vi "Change Baud or Unit ID.vi"(7 "Unit ID (A)":string="A", 8 "error in":errorcluster, 9 "Change Unit Baud Rate":enum8{"2400", "9600", "19200", "38400"}(ring)=enum."19200", 10 "Change Unit ID":i32(ring)=65 items=["@ (limit 1 streaming unit per port)"=64, "A"=65, "B"=66, "C"=67, "D"=68, "E"=69, "F"=70, "G"=71, "H"=72, "I"=73, "J"=74, "K"=75, "L"=76, "M"=77, "N"=78, "O"=79, "P"=80, "Q"=81, "R"=82, "S"=83, "T"=84, "U"=85, "V"=86, "W"=87, "X"=88, "Y"=89, "Z"=90], 11 "VISA Session In":refnum<visa-resource-name>="Alicat") -> (0 "error out":errorcluster, 3 "VISA Session Out":refnum<visa-resource-name>)   [LabVIEW 2016]
doc: "Changes the baud rate or the unit ID of an Alicat device."
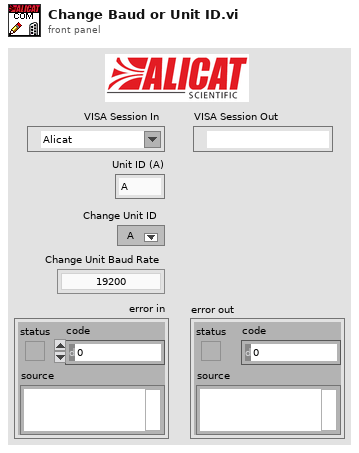
[diagram p1: front panel]
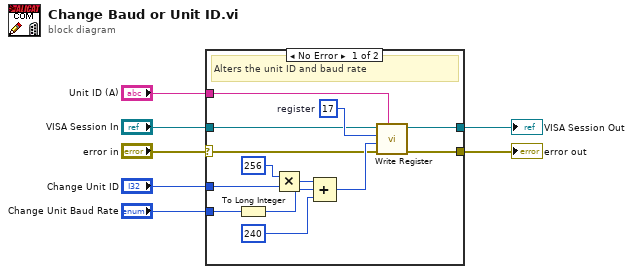
[diagram p0: block diagram]
diagram:
  n1 = case shown="No Error" "error in" {
    selector: "error in" -> [w8 w22]
    tunnel: "VISA Session In" -> [w19 w21]
    tunnel: "Unit ID (A)" -> [w18 _]
    tunnel: [w17 w21] -> w5
    tunnel: [w16 w22] -> w4
    tunnel: "Change Unit Baud Rate" -> [w15 _]
    tunnel: "Change Unit ID" -> [w11 _]
    frame No Error {
      w20 = u16 17  # register
      # "Alters the unit ID and baud rate"
      n2 = To Long Integer(number=w15) -> (32bit integer=w14:i32)
      n3 = Multiply(x=256 ("y"), y=w11) -> (x*y=w10:i32)
      n4 = Compound Arithmetic op=ADD(w10, w14, 240 ("y")) -> (w12:i32)
      n5 = call "Write Register.vi"("Unit ID (A)"=w18, "error in"=w8, "Register Value"=w12, "Register address"=w20, "VISA Session In"=w19) -> ("error out"=w16:errorcluster, "VISA Session Out"=w17:refnum<visa-resource-name>)  [unwired: 4 in, 1 out]
    }
    frame Error {
    }
  }
  "error out" <- w4
  "VISA Session Out" <- w5
